vi "Zadanie 1 v. 2.0..vi"() -> ()   [LabVIEW 2020]
panel:
  out "Array":dbl[](array[numeric])
  out "Liczba wygenerowana":dbl
  in  "stop":bool
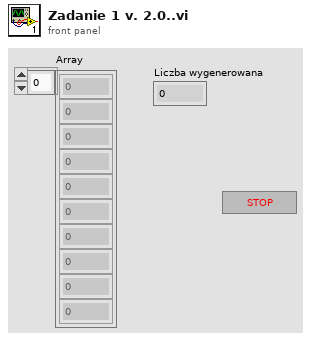
[diagram p1: front panel]
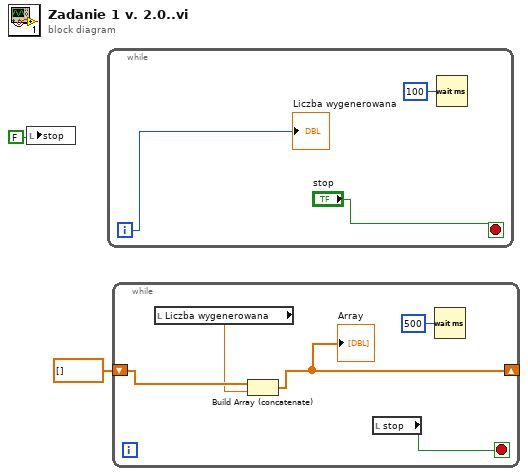
[diagram p0: block diagram]
diagram:
  n1 = local write "stop"(FALSE) -> ()
  n2 = while {
    i -> [w4]
    stop <- "stop" stop-if-true
    n3 = Wait (ms)(milliseconds to wait=u32 100) -> ()  [unwired: 1 out]
    "Liczba wygenerowana" <- w4
  }
  n4 = while {
    shift-right: [w7] -> _
    shift-left: dbl[] [] -> [w9]
    stop <- w10 stop-if-true
    n5 = local read "Liczba wygenerowana"() -> (w8:dbl)
    n6 = Build Array (concatenate)(w9, w8) -> (w7:dbl[])
    "Array" <- w7
    n7 = local read "stop"() -> (w10:bool)
    n8 = Wait (ms)(milliseconds to wait=u32 500) -> ()  [unwired: 1 out]
  }
